vi "Assign Heights.vi"(4 "Path on Command Branch Height":i32=35, 5 "Height Padding":i32, 6 "Leaf Height":i32=16, 7 "Default Path Height":i32=15, 8 "Command Height":i32=32, 9 "Leaf + Outcome Name Height":i32=38, 10 "Depth":i32, 11 "Tree with Depths in":T1) -> (2 "Max Height per Row":dbl[](array[numeric]), 3 "Tree with Heights Out":T1)   [LabVIEW 2025]
uses:
  Types/Decision Tree.ctl
  Types/Sequencing Tree Node.ctl
  Types/Single Cmd Info.ctl
  <vilib>/picture/picture.llb/imagedata.ctl
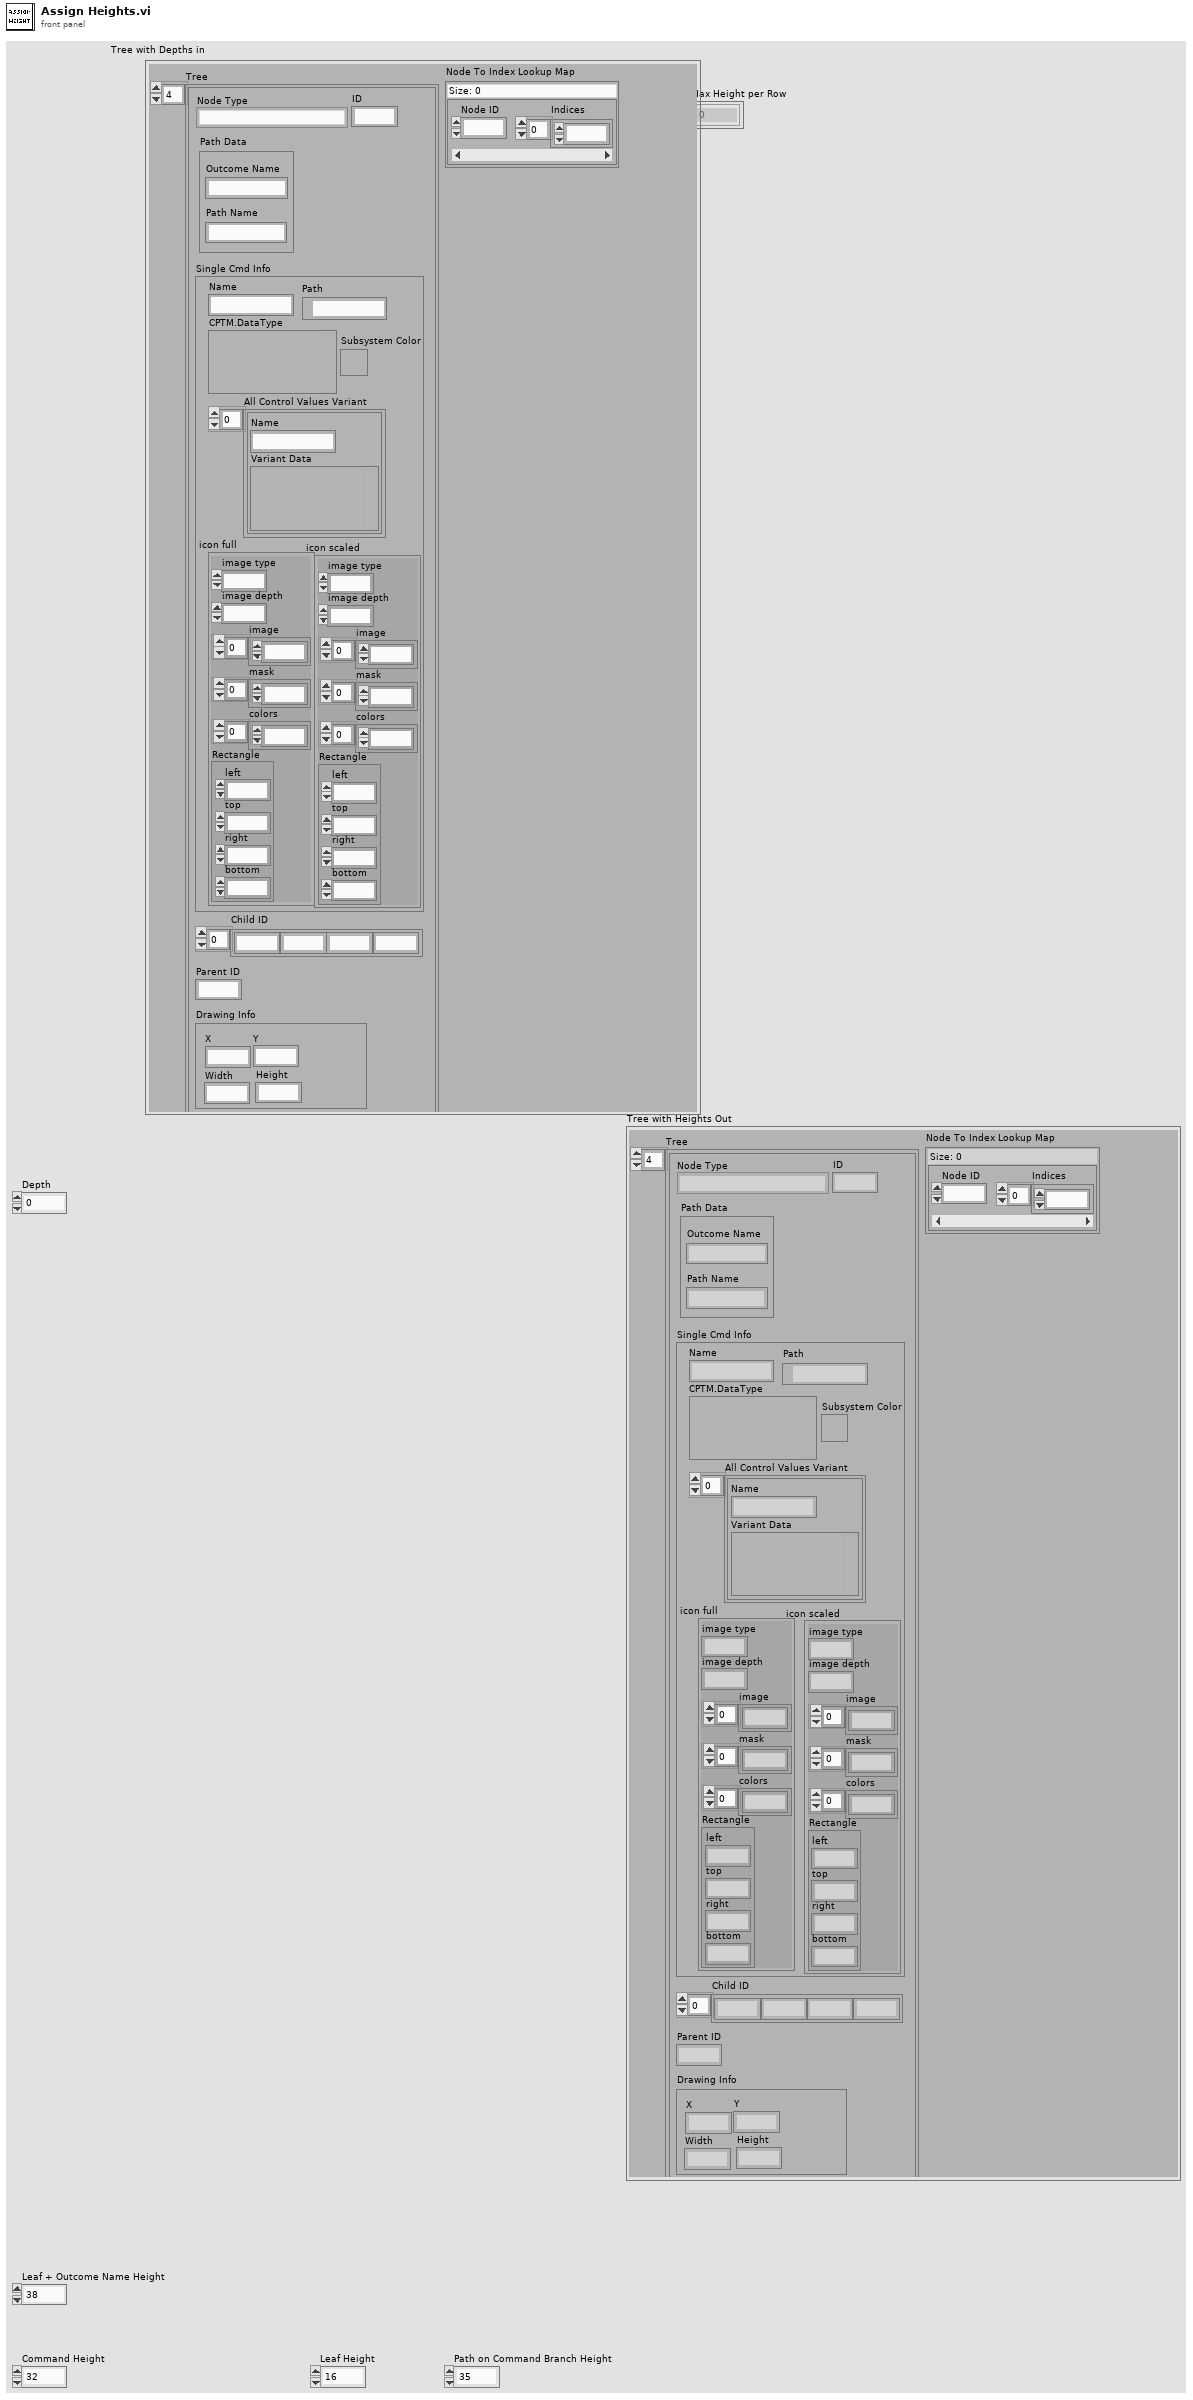
[diagram p1: front panel]
types:
  T1 = typedef "Decision Tree.ctl" = cluster{"Tree":T2[], "Node To Index Lookup Map":map{i16, i16[]}}
  T2 = typedef "Sequencing Tree Node.ctl" = cluster{"Node Type":enum16{"Path", "Command", "Leaf"}, "ID":i16, "Path Data":cluster{"Path Name":string, "Outcome Name":string}, "Single Cmd Info":T3, "Child ID":i32[], "Parent ID":i32, "Drawing Info":cluster{"X":i32, "Y":i32, "Width":i32, "Height":i32}}
  T3 = typedef "Single Cmd Info.ctl" = cluster{"Name":string, "CPTM.DataType":variant, "All Control Values Variant":cluster{"Name":string, "Variant Data":variant}[], "icon full":T4, "icon scaled":T4, "Path":path, "Subsystem Color":u32}
  T4 = typedef "imagedata.ctl" = cluster{"image type":i32, "image depth":i32, "image":u8[], "mask":u8[], "colors":u32[], "Rectangle":cluster{"left":i16, "top":i16, "right":i16, "bottom":i16}}
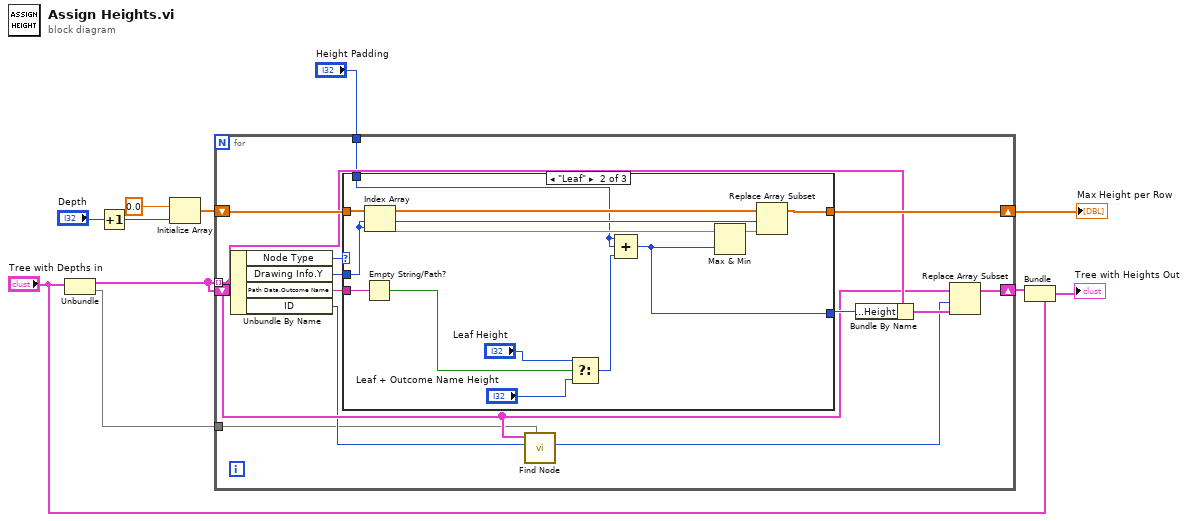
[diagram p0: block diagram]
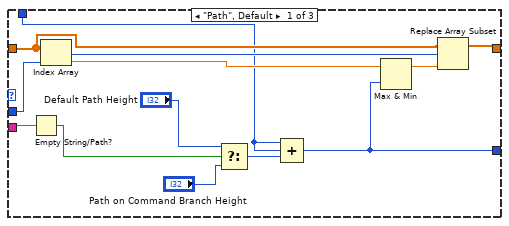
[diagram p2: hidden frame]
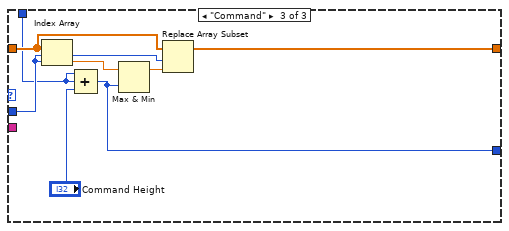
[diagram p3: hidden frame]
diagram:
  n1 = Unbundle("Tree with Depths in") -> ("Tree"=w5:T2[], "Node To Index Lookup Map"=w1:map{i16, i16[]})
  n2 = Increment(x="Depth") -> (x+1=w10:i32)
  n3 = Initialize Array(0.0, w10) -> (w8:dbl[])
  n4 = for {
    tunnel: w5 -> [w20] mode=indexing
    shift-right: [w22] -> w6
    shift-left: w8 -> [w23]
    shift-right: [w17] -> w4
    shift-left: w5 -> [w15]
    tunnel: "Height Padding" -> [w16]
    tunnel: w1 -> [w13]
    n5 = Unbundle By Name(w20) -> ("Node Type"=w25:enum16{"Path", "Command", "Leaf"}, "Drawing Info.Y"=w24:i32, "Path Data.Outcome Name"=w21:string, "ID"=w14:i16)
    n6 = case shown="\"Leaf\"" w25 {
      tunnel: w24 -> [w36 w49 w53]
      tunnel: w23 -> [w37 w48 w57]
      tunnel: [w35 w47 w56] -> w22
      tunnel: w21 -> [w34 w44 _]
      tunnel: [w27 w39 w51] -> w19
      tunnel: w16 -> [w26 w38 w50]
      frame "Path", Default {
        n7 = Empty String/Path?(string/path=w34) -> (empty?=w33:bool)
        n8 = Index Array(array=w37, index=w36) -> (element=w30:dbl)
        n9 = Select(t="Default Path Height", s=w33, f="Path on Command Branch Height") -> (s? t:f=w28:i32)
        n10 = Compound Arithmetic op=ADD(w26, w26, w28) -> (w27:i32)
        n11 = Max & Min(x=w30, y=w27) -> (max(x,y)=w29:dbl)  [unwired: 1 out]
        n12 = Replace Array Subset(array=w37, new element=w29, index=w36) -> (w35:dbl[])
      }
      frame "Leaf" {
        n13 = Empty String/Path?(string/path=w44) -> (empty?=w43:bool)
        n14 = Index Array(array=w48, index=w49) -> (element=w46:dbl)
        n15 = Select(t="Leaf Height", s=w43, f="Leaf + Outcome Name Height") -> (s? t:f=w40:i32)
        n16 = Compound Arithmetic op=ADD(w38, w38, w40) -> (w39:i32)
        n17 = Max & Min(x=w46, y=w39) -> (max(x,y)=w45:dbl)  [unwired: 1 out]
        n18 = Replace Array Subset(array=w48, new element=w45, index=w49) -> (w47:dbl[])
      }
      frame "Command" {
        n19 = Index Array(array=w57, index=w53) -> (element=w55:dbl)
        n20 = Compound Arithmetic op=ADD(w50, w50, "Command Height") -> (w51:i32)
        n21 = Max & Min(x=w55, y=w51) -> (max(x,y)=w54:dbl)  [unwired: 1 out]
        n22 = Replace Array Subset(array=w57, new element=w54, index=w53) -> (w56:dbl[])
      }
    }
    n23 = call "Find Node.vi"("Node To Index Lookup Map"=w13, "ID"=w14, "Tree"=w15) -> ("Index"=w12:i16)  [unwired: 7 in, 1 out]
    n24 = Bundle By Name(cluster=w20, "Drawing Info.Height"=w19) -> (w18:T2)
    n25 = Replace Array Subset(array=w15, new element=w18, index=w12) -> (w17:T2[])
  }
  "Max Height per Row" <- w6
  n26 = Bundle(cluster="Tree with Depths in", "Tree"=w4) -> (→"Tree with Heights Out":T1)  [unwired: 1 in]
